vi "ConvertWindowToDisplayWindowCommand.vi"(11 "Window":u8 min=1 max=2 step=1) -> (3 "Display Window Command":string)   [LabVIEW 2009, in "Keithley-6482-Visa.lvlib"]
uses:
  <instrlib>/Keithley-6482-Visa9.0/Keithley-6482-Visa.lvlib
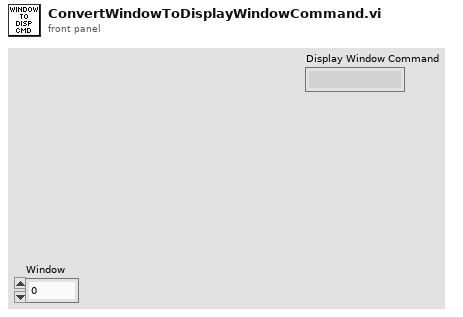
[diagram p1: front panel]
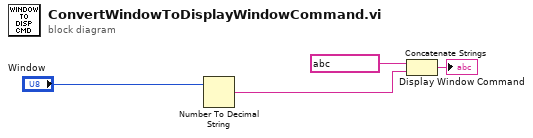
[diagram p0: block diagram]
diagram:
  n1 = Number To Decimal String(number="Window") -> (decimal integer string=w2:string)  [unwired: 1 in]
  n2 = Concatenate Strings(string ?, w2) -> (→"Display Window Command":string)
